vi "Module Loop.vi"(8 "error in (no error)":errorcluster, 11 "System Health Module in":refnum<class "System Health Module.lvclass">) -> (0 "error out":errorcluster, 3 "System Health Module out":refnum<class "System Health Module.lvclass">)   [LabVIEW 2020, in "Volatus.lvlib" / "System Health Module.lvclass"]
uses:
  System Health Module.lvclass
  C:/dev/lv20CE/relink/lv-volatus/Volatus/Module/Module.lvclass
  Module/Module.lvclass
  Module/Module.lvclass/Module.ctl
  <vilib>/Utility/error.llb/Error Cluster From Error Code.vi
  System Health Module.lvclass/System Health Module.ctl
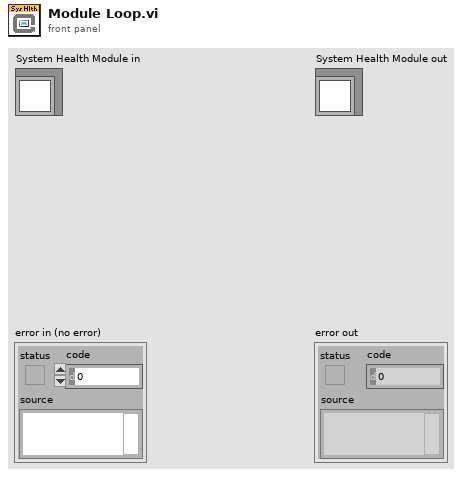
[diagram p1: front panel]
types:
  T1 = enum32{"Invalid", "Standard", "Closed", "Hidden", "Minimized", "Maximized"}
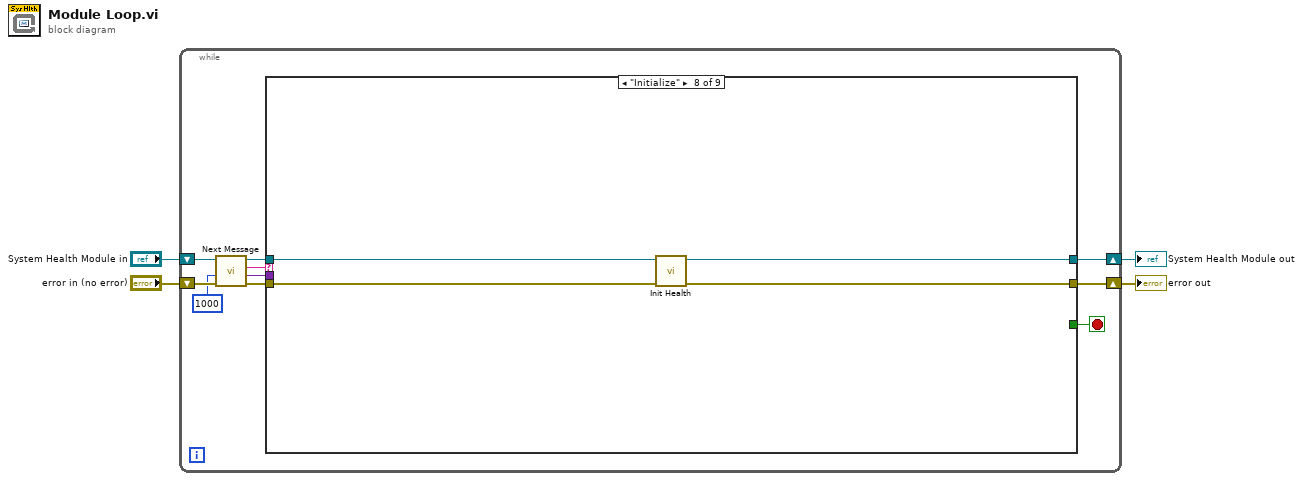
[diagram p0: block diagram]
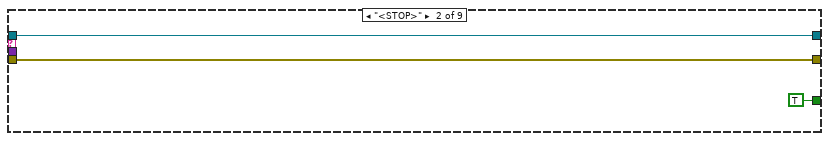
[diagram p3: hidden frame]
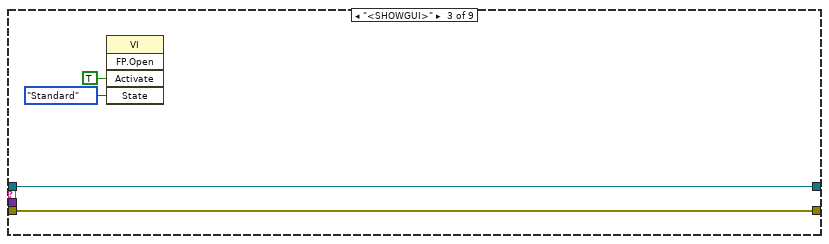
[diagram p4: hidden frame]
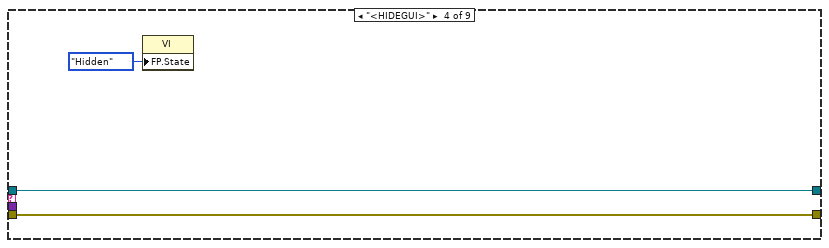
[diagram p5: hidden frame]
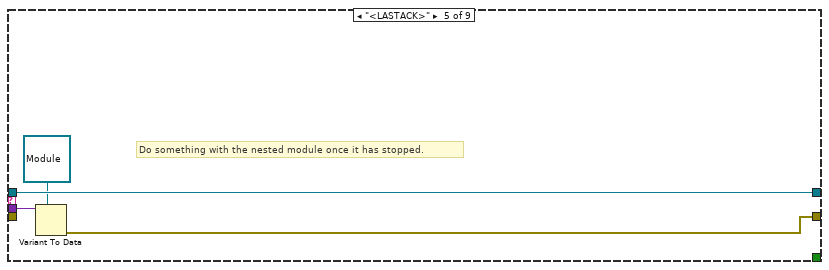
[diagram p6: hidden frame]
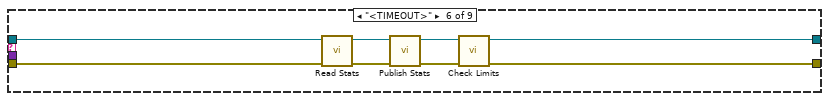
[diagram p7: hidden frame]
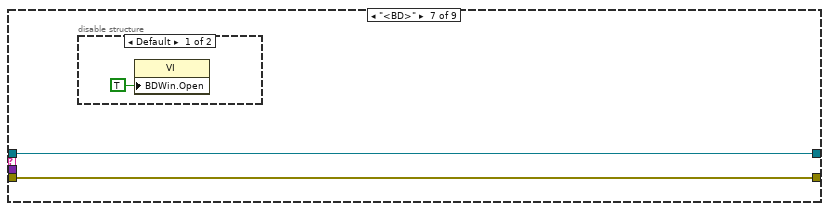
[diagram p8: hidden frame]
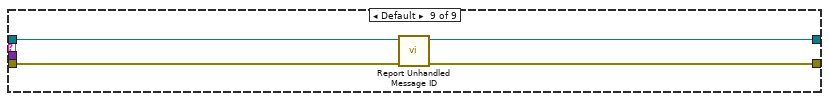
[diagram p10: hidden frame]
diagram:
  n1 = while {
    shift-right: [w9] -> w4
    shift-left: "System Health Module in" -> [w14]
    shift-right: [w8] -> w3
    shift-left: "error in (no error)" -> [w13]
    stop <- w7 stop-if-true
    n2 = call "Next Message.vi"("error in (no error)"=w13, "Timeout ms (-1)"=1000, "Module in"=w14) -> ("error out"=w12:errorcluster, "Data"=w6:variant, "ID"=w11:string, "Module out"=w10:refnum<class "System Health Module.lvclass">)  [unwired: 5 in]
    n3 = case shown="\"Initialize\"" w11 {
      tunnel: w12 -> [w15 w18 w22 w25 _ w33 w39 w45 w49]
      tunnel: w10 -> [w16 w19 w23 w26 w30 w34 w40 w43 w47]
      tunnel: [w16 w19 w23 w26 w30 w31 w40 w42 w46] -> w9
      tunnel: [w15 w18 w22 w25 w27 w32 w39 w44 w48] -> w8
      tunnel: [_ TRUE _ _ _ _ _ _ _] -> w7
      tunnel: w6 -> [_ _ _ _ w29 _ _ _ _]
      frame "<CLOSE>" {
      }
      frame "<STOP>" {
      }
      frame "<SHOWGUI>" {
        n4 = invoke class="VI" method="FP.Open"("Activate"=TRUE ("Activate?"), "State"=T1."Standard") -> ()  [unwired: 3 in, 5 out]
      }
      frame "<HIDEGUI>" {
        n5 = property class="VI"("FP.State"=T1."Hidden" ("Front Panel Window:State")) -> ()  [unwired: 2 in, 2 out]
      }
      frame "<LASTACK>" {
        # "Do something with the nested module once it has stopped."
        n6 = Variant To Data(type=refnum<class "Module.lvclass"> refnum ("Volatus:Module"), Variant=w29) -> (error out=w27:errorcluster)  [unwired: 1 in, 1 out]
      }
      frame "<TIMEOUT>" {
        n7 = call "Read Stats.vi"("error in (no error)"=w33, "System Health Module in"=w34) -> ("error out"=w38:errorcluster, "System Health Module out"=w36:refnum<class "System Health Module.lvclass">)  [unwired: 8 in]
        n8 = call "Publish Stats.vi"("error in (no error)"=w38, "System Health Module in"=w36) -> ("error out"=w37:errorcluster, "System Health Module out"=w35:refnum<class "System Health Module.lvclass">)  [unwired: 8 in]
        n9 = call "Check Limits.vi"("error in (no error)"=w37, "System Health Module in"=w35) -> ("error out"=w32:errorcluster, "System Health Module out"=w31:refnum<class "System Health Module.lvclass">)  [unwired: 8 in]
      }
      frame "<BD>" {
        n10 = disable-structure shown="Default" {
          frame condition #0 (active) {
            n11 = property class="VI"("BDWin.Open"=TRUE ("Block Diagram Window:Open")) -> ()  [unwired: 2 in, 2 out]
          }
          frame condition #1 {
          }
        }
      }
      frame "Initialize" {
        n12 = call "Init Health.vi"("error in (no error)"=w45, "System Health Module in"=w43) -> ("error out"=w44:errorcluster, "System Health Module out"=w42:refnum<class "System Health Module.lvclass">)  [unwired: 8 in]
      }
      frame Default {
        n13 = call "Report Unhandled Message ID.vi"("error in (no error)"=w49, "Module in"=w47) -> ("error out"=w48:errorcluster, "Module out"=w46:refnum<class "System Health Module.lvclass">)  [unwired: 8 in]
      }
    }
  }
  "error out" <- w3
  "System Health Module out" <- w4
